vi "StatusConnectedGuard.vi"(11 "error":errorcluster) -> (3 "EnableOut":bool)   [LabVIEW 2020]
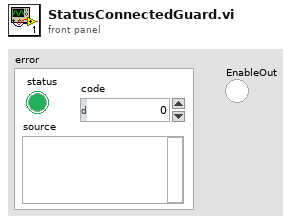
[diagram p1: front panel]
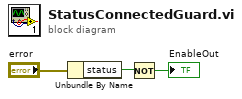
[diagram p0: block diagram]
diagram:
  n1 = Unbundle By Name("error") -> ("status"=w2:bool)
  n2 = Not(x=w2) -> (.not. x?=→"EnableOut":bool)
